vi "Write Prober INI File.vi"(0 "configuration file path":path=path "C:/Users/Eddie.Rickey/Documents/RCV_PXI/Prober Configuration File.ini", 1 "Prober INI  Key Value":string="False", 2 "Prober INI Key":string="Test Complete", 11 "Error In":errorcluster) -> (15 "Error Out":errorcluster)   [LabVIEW 2013]
uses:
  <vilib>/Utility/config.llb/Write Key (String).vi
  <vilib>/Utility/config.llb/NI_LVConfig.lvlib
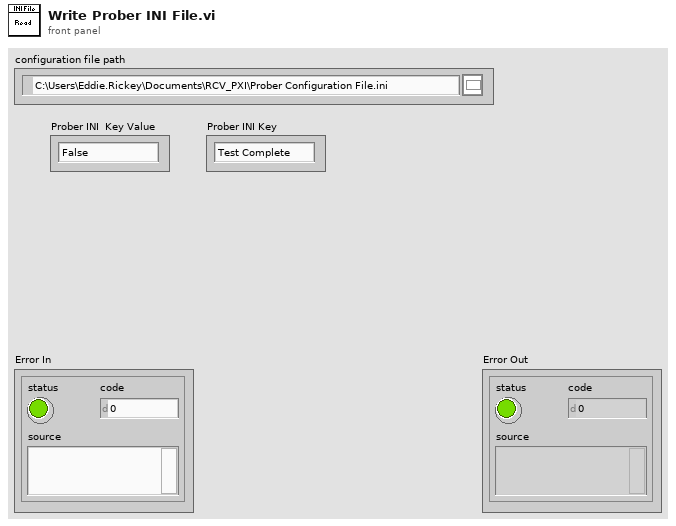
[diagram p1: front panel]
types:
  T1 = typedef "NI_LVConfig.lvlib/Config Data RefNum.ctl" = refnum<k1>
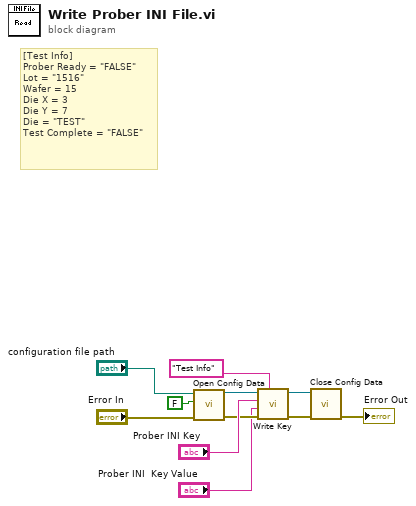
[diagram p0: block diagram]
diagram:
  # "[Test Info]\nProber Ready = \"FALSE\"\nLot = \"1516\"\nWafer = 15\nDie X = 3\nDie Y = 7\nDie = \"TEST\"\nTest Complete = \"FALSE\""
  n1 = call <vilib>:"Open Config Data.vi"("error in (no error)"="Error In", "create file if necessary (T)"=FALSE, "configuration file path"="configuration file path") -> ("error out"=w5:errorcluster, "refnum"=w4:T1)  [unwired: 6 in, 1 out]
  n2 = call-poly <vilib>:"Write Key.vi"("section"="Test Info", "error in (no error)"=w5, "value"="Prober INI  Key Value", "key"="Prober INI Key", "refnum"=w4) -> ("error out"=w3:errorcluster, "refnum out"=w2:T1)  [unwired: 4 in, 1 out]
  n3 = call <vilib>:"Close Config Data.vi"("error in (no error)"=w3, "refnum"=w2) -> ("error out"=→"Error Out":errorcluster)  [unwired: 8 in, 1 out]
